vi "Grafico_XY.vi"() -> ()   [LabVIEW 2016]
panel:
  out "Waveform Graph Y":dbl[](graph)
  out "Waveform Graph X":dbl[](graph)
  out "Tamano_X":i32
  out "XY Graph DAC":cluster{dbl[], dbl[]}(graph)
  out "Columnas":i32
  out "Filas":i32
  out "XY Graph":cluster{i32[], i32[]}(graph)
  out "Array 2":i32[](array[numeric])
  out "Array":i32[](array[numeric])
  out "1-bit pixmap":bool[][](array[boolean])
  out "Logotipo":picture
  in  "File Path":path
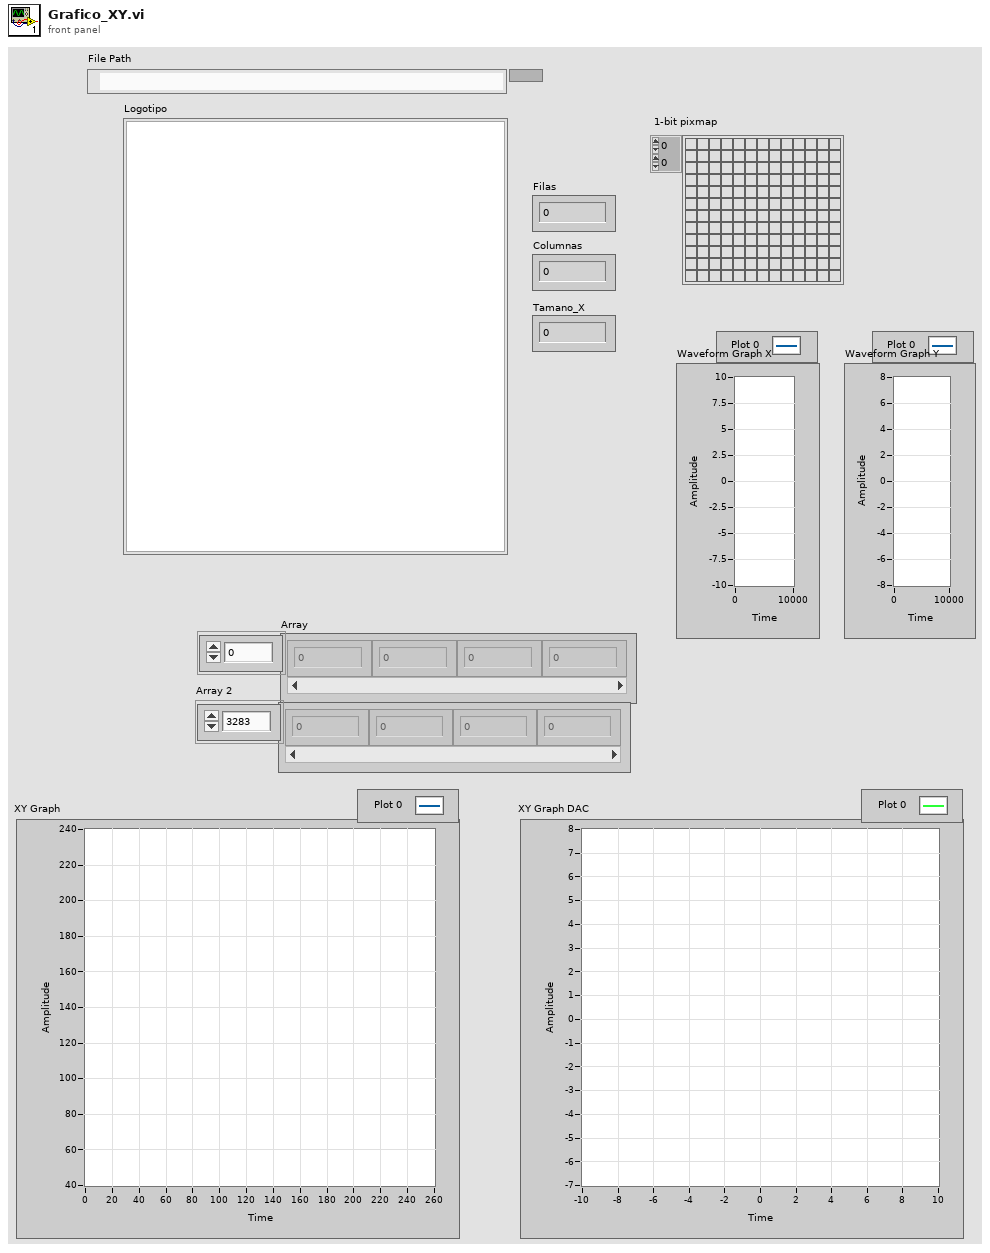
[diagram p1: front panel]
types:
  T1 = typedef "imagedata.ctl" = cluster{"image type":i32, "image depth":i32, "image":u8[], "mask":u8[], "colors":u32[], "Rectangle":cluster{"left":i16, "top":i16, "right":i16, "bottom":i16}}
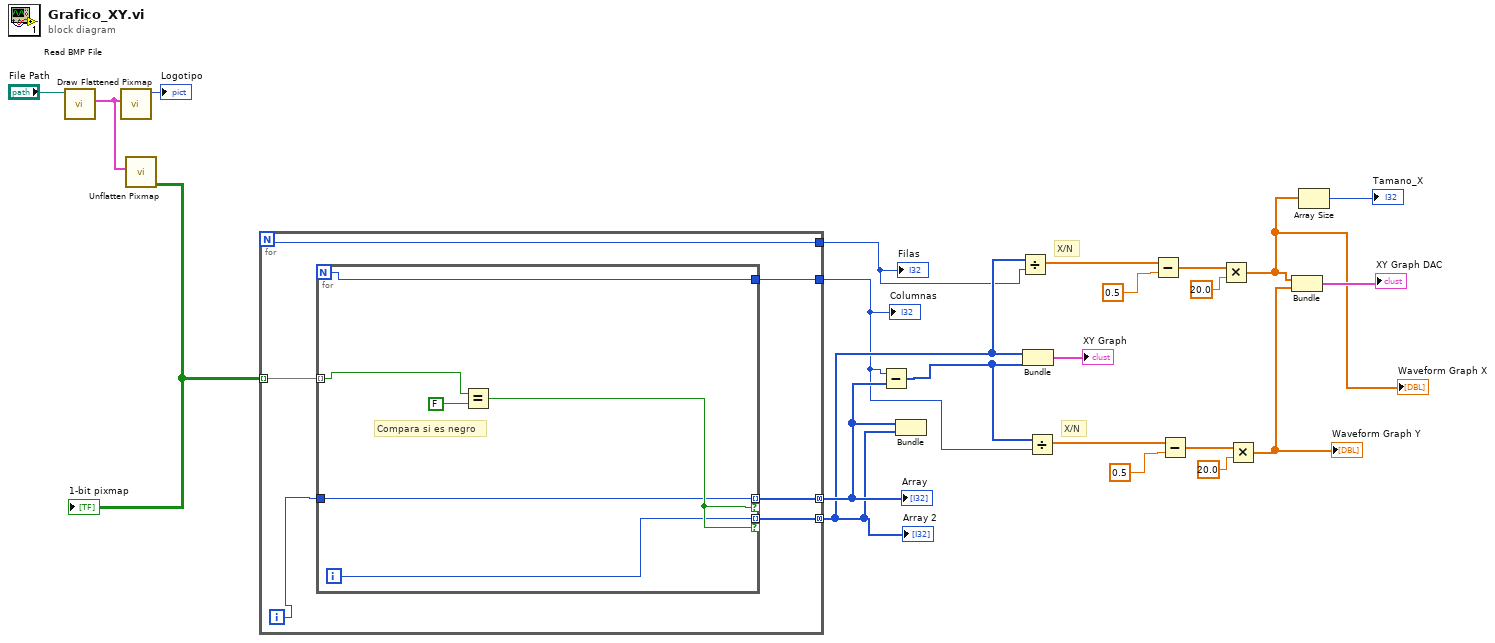
[diagram p0: block diagram]
diagram:
  # "X/N"
  # "X/N"
  n1 = call <vilib>:"Read BMP File.vi"("path to BMP file"="File Path") -> ("image data"=w20:T1)  [unwired: 8 in, 2 out]
  n2 = call <vilib>:"Draw Flattened Pixmap.vi"("image data"=w20) -> ("new picture"=→"Logotipo":picture)  [unwired: 8 in]
  n3 = call <vilib>:"Unflatten Pixmap.vi"("image data"=w20) -> ("1-bit pixmap"=w19:bool[][])  [unwired: 4 in, 6 out]
  "1-bit pixmap" <- w19
  n4 = for {
    N -> [w24]
    tunnel: w19 -> [w28] mode=indexing
    tunnel: [w26] -> w18 mode=concatenating
    tunnel: [w25] -> w16 mode=concatenating
    tunnel: [w24] -> w15
    tunnel: [w23] -> w4
    i -> [w27]
    n5 = for {
      N -> [w29]
      tunnel: w28 -> [w34] mode=indexing
      tunnel: w27 -> [w31]
      tunnel: [w30] -> w25 mode=indexing if=w32
      tunnel: [w31] -> w26 mode=indexing if=w32
      tunnel: [w29] -> w23
      i -> [w30]
      # "Compara si es negro"
      n6 = Equal?(x=w34, y=FALSE) -> (x = y?=w32:bool)
    }
  }
  "Array" <- w18
  "Array 2" <- w16
  "Filas" <- w15
  "Columnas" <- w4
  n7 = Subtract(x=w4, y=w18) -> (x-y=w5:i32[])
  n8 = Bundle(w18, w16) -> ()  [unwired: 1 in, 1 out]
  n9 = Divide(x=w16, y=w15) -> (x/y=w14:dbl[])
  n10 = Bundle(w16, w5) -> (→"XY Graph":cluster{i32[], i32[]})  [unwired: 1 in]
  n11 = Divide(x=w5, y=w4) -> (x/y=w9:dbl[])
  n12 = Subtract(x=w14, y=0.5) -> (x-y=w12:dbl[])
  n13 = Subtract(x=w9, y=0.5) -> (x-y=w7:dbl[])
  n14 = Multiply(x=w12, y=20.0) -> (x*y=w2:dbl[])
  "Waveform Graph X" <- w2
  n15 = Multiply(x=w7, y=20.0) -> (x*y=w1:dbl[])
  "Waveform Graph Y" <- w1
  n16 = Bundle "Bundle"(w2, w1) -> (→"XY Graph DAC":cluster{dbl[], dbl[]})  [unwired: 1 in]
  n17 = Array Size(array=w2) -> (size(s)=→"Tamano_X":i32)
